vi "PH_BeamlineInformation.PC _Voltage of Head.vi"(0 "i ref in":refnum<vi>, 2 "Voltage Service Name":string, 3 "Voltage [V]":dbl, 4 "no link?":bool, 5 "error in (no error)":errorcluster) -> (14 "i ref out":refnum<vi>, 19 "error out":errorcluster)   [LabVIEW 2014, in "PH_BeamlineInformation.lvlib"]
doc: "This VI writes the incoming information (if changed) to own attributes."
uses:
  PH_BeamlineInformation.lvlib
  PH_Common/PH_Common.lvlib
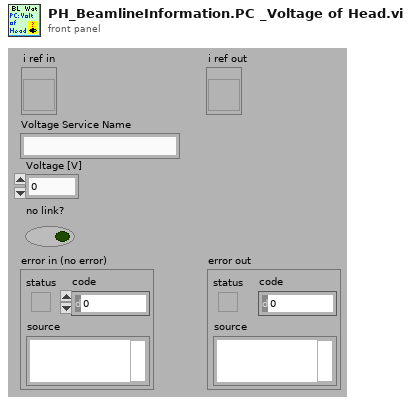
[diagram p1: front panel]
types:
  T1 = enum8{"Enabled", "Disabled", "Disabled and Grayed Out"}
  T2 = typedef "PH_BeamlineInformation.lvlib/PH_BeamlineInformation.i attribute.ctl" = cluster{"BL GUI Elements of Services":cluster{"Service Name":string, "GUI Elements":refnum<vi>[], "Status":i32}[], "Powermeters":T3, "Efficiency":T4, "Heads":T5[]}
  T3 = typedef "PH_BeamlineInformation.lvlib/PH_BeamlineInformation.Powermeter.ctl" = cluster{"ns FE":cluster{"GUI Ref":refnum<vi>, "Value":dbl}, "fs FE":cluster{"GUI Ref":refnum<vi>, "Value":dbl}, "PA":cluster{"GUI Ref":refnum<vi>, "Value":dbl}, "MA":cluster{"GUI Ref":refnum<vi>, "Value":dbl}, "Z6 green":cluster{"GUI Ref":refnum<vi>, "Value":dbl}, "Z6 IR":cluster{"GUI Ref":refnum<vi>, "Value":dbl}, "Z6 COS":cluster{"GUI Ref":refnum<vi>, "Value":dbl}}
  T4 = typedef "PH_BeamlineInformation.lvlib/PH_BeamlineInformation.Efficiency.ctl" = cluster{"PA Gain":cluster{"GUI Ref":refnum<vi>, "Value":dbl}, "MA Gain":cluster{"GUI Ref":refnum<vi>, "Value":dbl}, "Z6 green Conversion":cluster{"GUI Ref":refnum<vi>, "Value":dbl}, "Z6 Comp Losses":cluster{"GUI Ref":refnum<vi>, "Value":dbl}}
  T5 = typedef "PH_BeamlineInformation.lvlib/PH_BeamlineInformation.Head.ctl" = cluster{"PowerUnit":T6, "in use":cluster{"Value":bool, "GUI Ref":refnum<vi>, "linked":bool}, "voltage":cluster{"Value":dbl, "GUI Ref":refnum<vi>, "linked":bool}}
  T6 = typedef "PH_PP_Common.lvlib/PH_PP_Common.PUs.ctl" = enum16{"no Info", "PA-19mm-1", "PA-19mm-2", "PA-45mm-PILC", "PA-45mm-MAIN", "MA-PU-1", "MA-PU-2", "MA-PU-3", "MA-PU-4", "MA-PU-5", "MA-PU-6", "MA-FR", "MA-PILC", "PA-45mm-DP"}
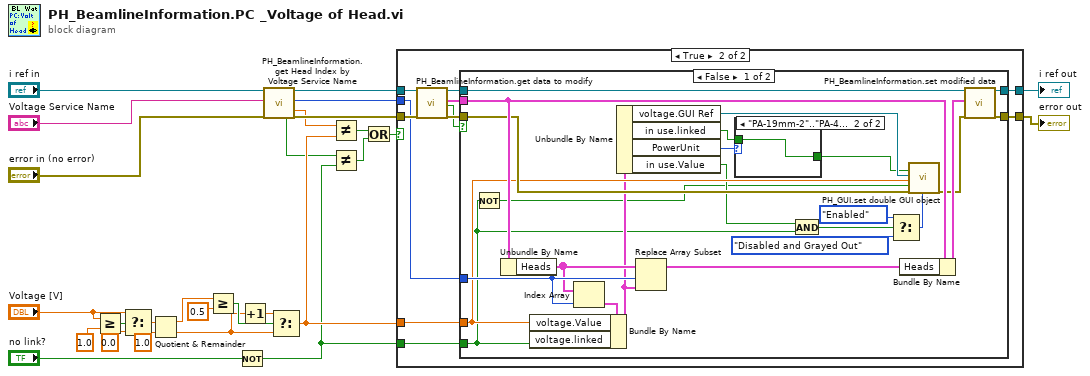
[diagram p0: block diagram]
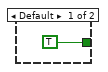
[diagram p3: hidden frame]
diagram:
  n1 = Greater Or Equal?(x="Voltage [V]", y=1.0) -> (x >= y?=w17:bool)
  n2 = Select(t="Voltage [V]", s=w17, f=0.0) -> (s? t:f=w15:dbl)
  n3 = Quotient & Remainder(x=w15, y=1.0) -> (x-y*floor(x/y)=w13:dbl, floor(x/y)=w10:dbl)
  n4 = Greater Or Equal?(x=w13, y=0.5) -> (x >= y?=w11:bool)
  n5 = Not(x="no link?") -> (.not. x?=w2:bool)
  n6 = Increment(x=w10) -> (x+1=w9:dbl)
  n7 = call "PH_BeamlineInformation.get Head Index by Voltage Service Name.vi"("i ref in"="i ref in", "Voltage Service Name"="Voltage Service Name", "error in (no error)"="error in (no error)") -> ("Voltage linked?"=w6:bool, "i ref out"=w22:refnum<vi>, "index of element"=w20:i32, "Voltage [V]"=w24:dbl, "error out"=w25:errorcluster)  [unwired: 11 in, 1 out]
  n8 = Select(t=w9, s=w11, f=w10) -> (s? t:f=w7:dbl)
  n9 = Not Equal?(x=w24, y=w7) -> (x != y?=w23:bool)
  n10 = Not Equal?(x=w6, y=w2) -> (x != y?=w4:bool)
  n11 = Or(x=w23, y=w4) -> (x .or. y?=w5:bool)
  n12 = case shown="True" w5 {
    tunnel: w25 -> [w29 w40]
    tunnel: w7 -> [_ w39]
    tunnel: [w29 w37] -> w1
    tunnel: w22 -> [w28 w36]
    tunnel: [w28 w34] -> w21
    tunnel: w20 -> [_ w31]
    tunnel: w2 -> [_ w30]
    frame False {
    }
    frame True {
      n13 = call "PH_BeamlineInformation.get data to modify.vi"("i ref in"=w36, "error in (no error)"=w40) -> ("i ref out"=w35:refnum<vi>, "i attribute"=w33:T2, "timed out"=w32:bool, "error out"=w38:errorcluster)  [unwired: 14 in]
      n14 = case shown="False" w32 {
        tunnel: w39 -> [w52 _]
        tunnel: w38 -> [w55 w67]
        tunnel: [w64 w67] -> w37
        tunnel: w35 -> [w63 w68]
        tunnel: [w62 w68] -> w34
        tunnel: w33 -> [w60 _]
        tunnel: w31 -> [w58 _]
        tunnel: w30 -> [w42 _]
        frame False {
          n15 = Not(x=w42) -> (.not. x?=w43:bool)
          n16 = Unbundle By Name(w60) -> ("Heads"=w57:T5[])
          n17 = Index Array(array=w57, index=w58) -> (element=w59:T5)
          n18 = Bundle By Name(cluster=w59, "voltage.Value"=w52, "voltage.linked"=w42) -> (w46:T5)
          n19 = Unbundle By Name(w46) -> ("voltage.GUI Ref"=w53:refnum<vi>, "in use.linked"=w41:bool, "PowerUnit"=w45:T6, "in use.Value"=w51:bool)
          n20 = Replace Array Subset(array=w57, new element=w46, index=w58) -> (w56:T5[])
          n21 = case shown="\"PA-19mm-2\"..\"PA-45mm-MAIN\"" w45 {
            tunnel: [TRUE w66] -> w44
            tunnel: w41 -> [_ w66]
            frame Default {
            }
            frame "PA-19mm-2".."PA-45mm-MAIN" {
            }
          }
          n22 = And(x=w51, y=w42) -> (x .and. y?=w50:bool)
          n23 = Select(t=T1."Enabled" ("Disabled (Enabled)"), s=w50, f=T1."Disabled and Grayed Out") -> (s? t:f=w48:T1)
          n24 = Bundle By Name(cluster=w60, "Heads"=w56) -> (w61:T2)
          n25 = call "PH_GUI.set double GUI object.vi"("visible (true)"=w44, "GUI object Ref"=w53, "value"=w52, "blinking (false)"=w43, "error in (no error)"=w55, "Disabled (Enabled)"=w48) -> ("error out"=w54:errorcluster)  [unwired: 13 in]
          n26 = call "PH_BeamlineInformation.set modified data.vi"("i ref in"=w63, "i attribute"=w61, "error in (no error)"=w54) -> ("i ref out"=w62:refnum<vi>, "error out"=w64:errorcluster)  [unwired: 15 in]
        }
        frame True {
        }
      }
    }
  }
  "error out" <- w1
  "i ref out" <- w21
